vi "Active Cell Cell Size Separator.vi"(8 "error in (no error)":errorcluster, 10 "Boolean":bool, 11 "Tree in":refnum<class "TreeControl.lvclass">) -> (0 "error out":errorcluster, 3 "Tree out":refnum<class "TreeControl.lvclass">)   [LabVIEW 2015, in "TreeControl.lvclass"]
uses:
  TreeControl.lvclass
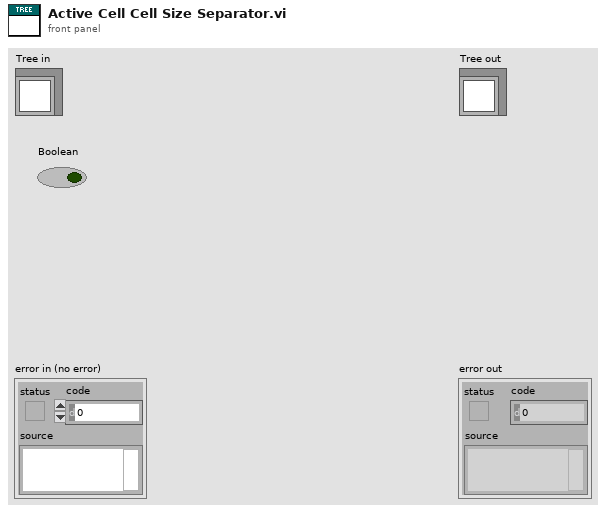
[diagram p1: front panel]
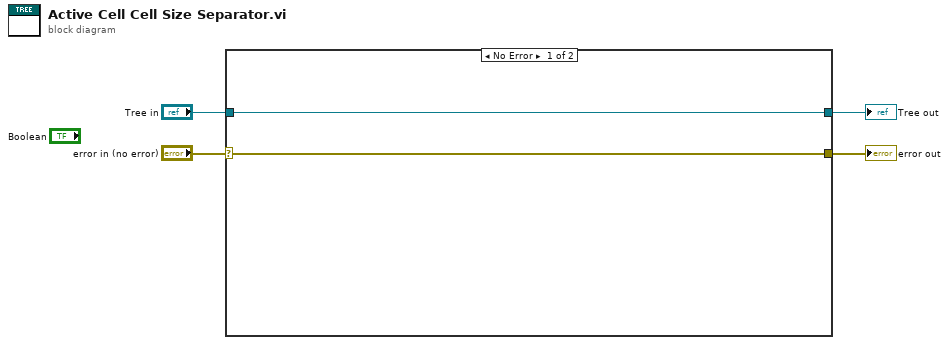
[diagram p0: block diagram]
diagram:
  n1 = case shown="No Error" "error in (no error)" {
    selector: "error in (no error)" -> [w5 w8]
    tunnel: [w5 w8] -> w3
    tunnel: [w6 w7] -> w1
    tunnel: "Tree in" -> [w6 w7]
    frame No Error {
    }
    frame Error {
    }
  }
  "error out" <- w3
  "Tree out" <- w1
